vi "terminate.vi"(8 "error in (no error)":errorcluster, 11 "GenericPlugin in":refnum<class "GenericScanHead.lvclass">) -> (0 "error out":errorcluster, 3 "GenericPlugin out":refnum<class "GenericScanHead.lvclass">)   [LabVIEW 2010, in "GenericScanHead.lvclass"]
doc: "The dynamic dispatch version of this VI terminates the plug-in object by releasing all of its resources."
uses:
  GenericScanHead.lvclass
  Trajectory/GenericTrajectory/GenericTrajectory/GenericTrajectory.lvclass
  common/classes/GenericToplevelComponent/GenericToplevelComponent/GenericToplevelComponent.lvclass
  common/classes/ErrorController/ErrorController/class_data.vi
  common/classes/ErrorController/ErrorController/ErrorController.lvclass
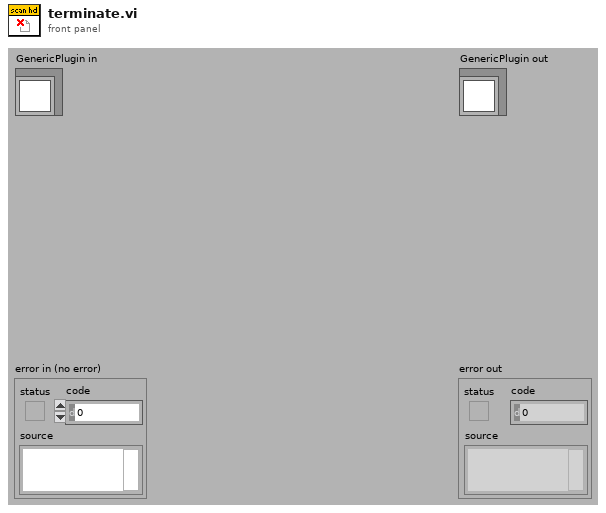
[diagram p1: front panel]
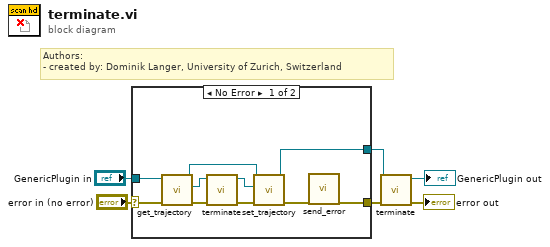
[diagram p0: block diagram]
diagram:
  # "Authors: \n- created by: Dominik Langer, University of Zurich, Switzerland"
  n1 = case shown="No Error" "error in (no error)" {
    selector: "error in (no error)" -> [w9 w18]
    tunnel: "GenericPlugin in" -> [w10 w17]
    tunnel: [w7 w18] -> w2
    tunnel: [w11 w17] -> w1
    frame No Error {
      n2 = call-dynamic "get_trajectory.vi"("error in (no error)"=w9, "GenericScanHead.lvclass in"=w10) -> ("error out"=w13:errorcluster, "trajectory"=w12:refnum<class "GenericTrajectory.lvclass">, "GenericScanHead.lvclass out"=w16:refnum<class "GenericScanHead.lvclass">)  [unwired: 7 in]
      n3 = call-dynamic "terminate.vi"("error in (no error)"=w13, "GenericPlugin in"=w12) -> ("error out"=w14:errorcluster, "GenericPlugin out"=w15:refnum<class "GenericTrajectory.lvclass">)  [unwired: 8 in]
      n4 = call-dynamic "set_trajectory.vi"("error in (no error)"=w14, "trajectory"=w15, "GenericScanHead.lvclass in"=w16) -> ("error out"=w8:errorcluster, "GenericScanHead.lvclass out"=w11:refnum<class "GenericScanHead.lvclass">)  [unwired: 7 in]
      n5 = call "send_error.vi"("error in (no error)"=w8) -> ("error out"=w7:errorcluster)  [unwired: 10 in]
    }
    frame Error {
    }
  }
  n6 = call-parent "terminate.vi"("error in (no error)"=w2, "GenericPlugin in"=w1) -> ("error out"=→"error out":errorcluster, "GenericPlugin out"=→"GenericPlugin out":refnum<class "GenericScanHead.lvclass">)  [unwired: 8 in]
